vi "Close.vi"(8 "error in (no error)":errorcluster, 11 "Hioki BT4560B":refnum<class "Hioki BT4560B.lvclass">) -> (0 "error out":errorcluster, 3 "Hioki BT4560B":refnum<class "Hioki BT4560B.lvclass">)   [LabVIEW 2019, in "Concrete.lvlib" / "Hioki BT4560B.lvclass"]
uses:
  Hioki BT4560B.lvclass
  Hioki BT4560B.lvclass/Hioki BT4560B.ctl
  Harware Abstraction/Analog In/Analog In.lvclass
  <instrlib>/HIOKI BT4560/HIOKI BT4560.lvlib
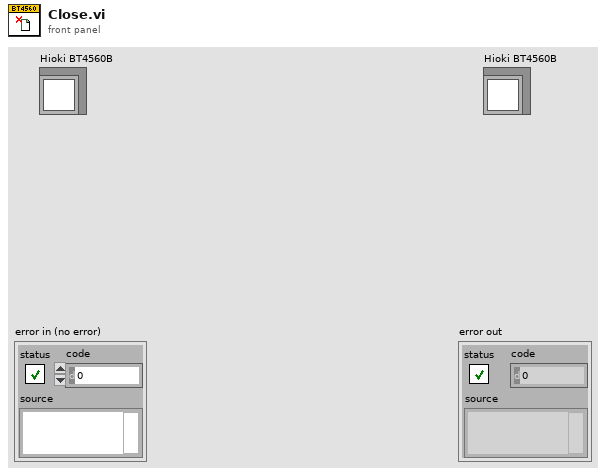
[diagram p1: front panel]
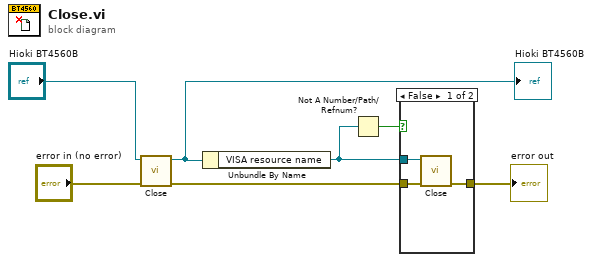
[diagram p0: block diagram]
diagram:
  n1 = call-parent <instrlib>:"Close.vi"("error in (no error)"="error in (no error)", "Instrument in"="Hioki BT4560B") -> ("error out"=w6:errorcluster, "Instrument out"=w1:refnum<class "Hioki BT4560B.lvclass">)  [unwired: 8 in]
  "Hioki BT4560B" <- w1
  n2 = Unbundle By Name(w1) -> ("VISA resource name"=w4:refnum<visa-resource-name>)
  n3 = Not A Number/Path/Refnum?(number/path/refnum=w4) -> (NaN/Path/Refnum?=w3:bool)
  n4 = case shown="False" w3 {
    tunnel: w6 -> [w10 w11]
    tunnel: [w8 w11] -> w5
    tunnel: w4 -> [w9 _]
    frame False {
      n5 = call <instrlib>:"Close.vi"("error in (no error)"=w10, "VISA resource name"=w9) -> ("error out"=w8:errorcluster)  [unwired: 9 in]
    }
    frame True {
    }
  }
  "error out" <- w5
